vi "Example.vi"(8 "error in (no error)":errorcluster, 11 "Path to JSON Sequence":path) -> (0 "error out":errorcluster)   [LabVIEW 2023, in "Easy.SequenceManagerLabVIEW.lvlib"]
uses:
  Easy.SequenceManagerLabVIEW.lvlib
  SequenceManager/SequenceManager.lvclass
  Parameter/Parameter.lvclass
  Step/Step.lvclass
panel:
  # "View block diagram\n for an explanation of this example"
  # "Connector Pane"
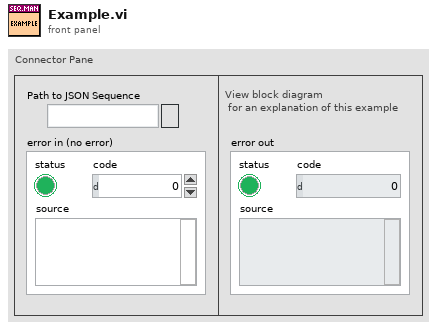
[diagram p1: front panel]
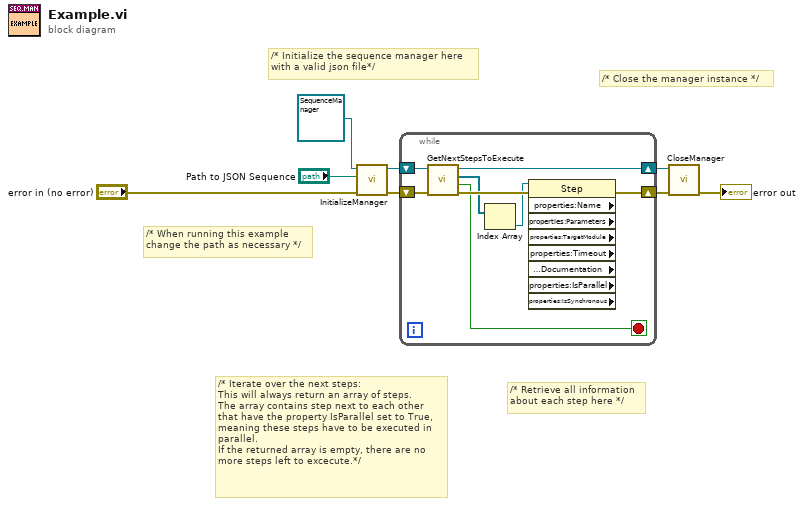
[diagram p0: block diagram]
diagram:
  # "/* When running this example\nchange the path as necessary */"
  # "/* Close the manager instance */"
  # "/* Retrieve all information\nabout each step here */"
  # "/* Iterate over the next steps:\nThis will always return an array of steps.\nThe array contains step next to each other \nthat have the property IsParallel set to True,\nmeaning these steps have to be executed in\nparallel.\nIf the returned array is empty, there are no\nmore steps left to excecute.*/"
  # "/* Initialize the sequence manager here \nwith a valid json file*/"
  n1 = call-dynamic "InitializeManager.vi"("error in (no error)"="error in (no error)", "Path to JSON sequence file"="Path to JSON Sequence", "SequenceManager in"=refnum<class "SequenceManager.lvclass"> refnum) -> ("error out"=w6:errorcluster, "SequenceManager out"=w3:refnum<class "SequenceManager.lvclass">)  [unwired: 7 in]
  n2 = while {
    shift-right: [w14] -> w5
    shift-left: w6 -> [w16]
    shift-right: [w12] -> w2
    shift-left: w3 -> [w13]
    stop <- w9 stop-if-true
    n3 = call-dynamic "GetNextStepsToExecute.vi"("error in (no error)"=w16, "SequenceManager in"=w13) -> ("error out"=w15:errorcluster, "Empty Array?"=w9:bool, "Steps"=w11:refnum<class "Step.lvclass">[], "SequenceManager out"=w12:refnum<class "SequenceManager.lvclass">)  [unwired: 6 in]
    n4 = Index Array(array=w11) -> (element=w10:refnum<class "Step.lvclass">)  [unwired: 1 in]
    n5 = property class="Step" props=["properties:Name", "properties:Parameters", "properties:TargetModule", "properties:Timeout", "properties:Documentation", "properties:IsParallel", "properties:IsSynchronous"](reference=w10, error in=w15) -> (error out=w14:errorcluster)  [unwired: 8 out]
  }
  n6 = call-dynamic "CloseManager.vi"("error in (no error)"=w5, "SequenceManager in"=w2) -> ("error out"=→"error out":errorcluster)  [unwired: 8 in, 1 out]
